vi "CRYRead License File.vi"(0 "License File Name":path) -> (12 "Public Key":u8[](array[numeric]) format="%x", 13 "License Key":u8[](array[numeric]) format="%x", 14 "error out":errorcluster, 16 "Data 1":u16 format="%x", 17 "Data 2":u16 format="%x", 18 "Data 3":u16 format="%x", 19 "Data 4":u16 format="%x")   [LabVIEW 2013]
panel:
  out "element 2":u8
  out "element":u8
  out "(hi.lo)":u16
  in  "error out":errorcluster
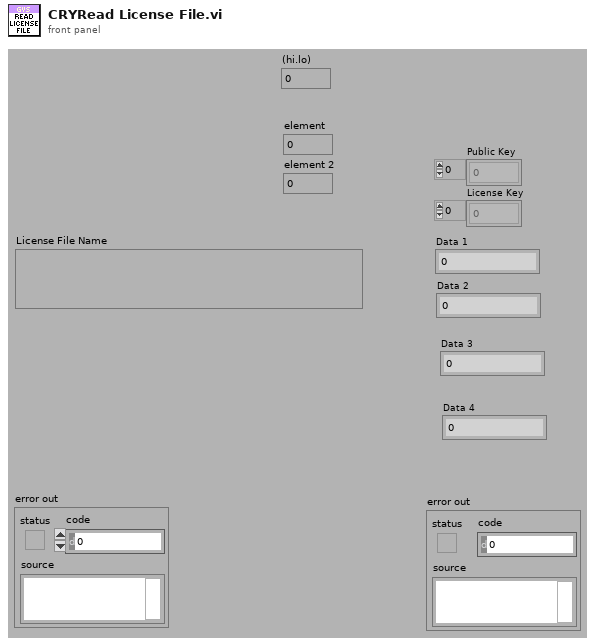
[diagram p1: front panel]
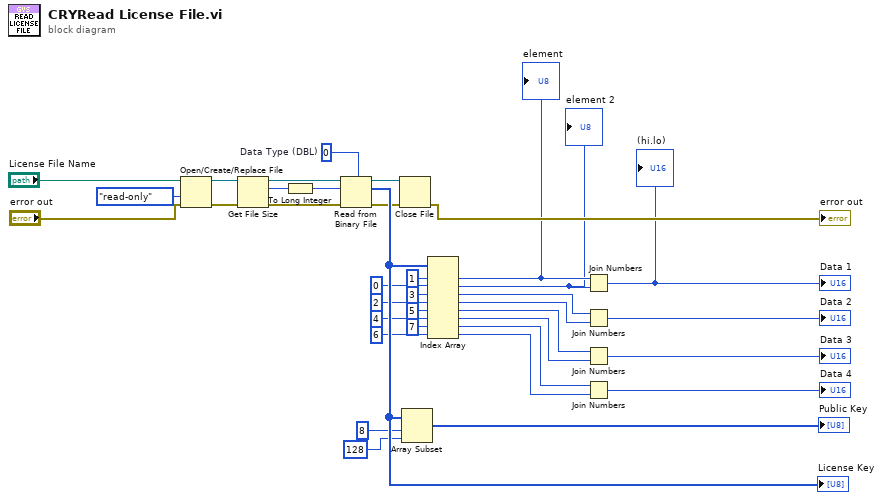
[diagram p0: block diagram]
diagram:
  w19 = u8 0  # Data Type (DBL)
  n1 = Open/Create/Replace File(file path (use dialog)="License File Name", error in="error out", access (0:read/write)=enum16{"read/write", "read-only", "write-only"}."read-only") -> (refnum out=w22:refnum<file>, error out=w21:errorcluster)  [unwired: 1 in, 3 out]
  n2 = Get File Size(file=w22, error in=w21) -> (refnum out=w25:refnum<file>, size (in bytes)=w24:i64, 0:w26:errorcluster)
  n3 = To Long Integer(number=w24) -> (32bit integer=w23:i32)
  n4 = Read from Binary File(5:w19, 8:w26, 10:w23, 11:w25) -> (0:w28:errorcluster, 2:w31:u8[], 3:w27:refnum<file>)  [unwired: 3 out]
  "License Key" <- w31
  n5 = Close File(refnum=w27, error in=w28) -> (error out=→"error out":errorcluster)  [unwired: 1 out]
  n6 = Array Subset(array=w31, index=8, length=128) -> (→"Public Key":u8[])
  n7 = Index Array(array=w31, index #1=1 ("index"), index #2=0 ("index"), index #3=3 ("index"), index #4=2 ("index"), index #5=5 ("index"), index #6=4 ("index"), index #7=7 ("index"), index #8=6 ("index")) -> (element #1=w10:u8, element #2=w9:u8, element #3=w8:u8, element #4=w7:u8, element #5=w6:u8, element #6=w5:u8, element #7=w4:u8, element #8=w3:u8)
  "element" <- w10
  "element 2" <- w9
  n8 = Join Numbers(hi=w10, lo=w9) -> ((hi.lo)=→"Data 1" →"(hi.lo)":u16)
  n9 = Join Numbers(hi=w8, lo=w7) -> ((hi.lo)=→"Data 2":u16)
  n10 = Join Numbers(hi=w6, lo=w5) -> ((hi.lo)=→"Data 3":u16)
  n11 = Join Numbers(hi=w4, lo=w3) -> ((hi.lo)=→"Data 4":u16)
